vi "FP_Move Window to Control Location.vi"(8 "Error":errorcluster, 9 "Vi To Move Settings":T2={"Menu Bar"=FALSE, "Position"=enum."MID-CTR", "Decoration index"=0, "border(px)"=-2, "Point"={"Left"=0, "Top"=0}}, 10 "Point":T1, 11 "VI To Move":refnum<vi>) -> (0 "Error Out":errorcluster)   [LabVIEW 2020]
uses:
  TypeDefs_Utility/Cluster_FP on Point Set.ctl
  TypeDefs_Utility/ENUM RB_Pos_Quadrant Position.ctl
  TypeDefs_Utility/Cluster_Top Left position.ctl
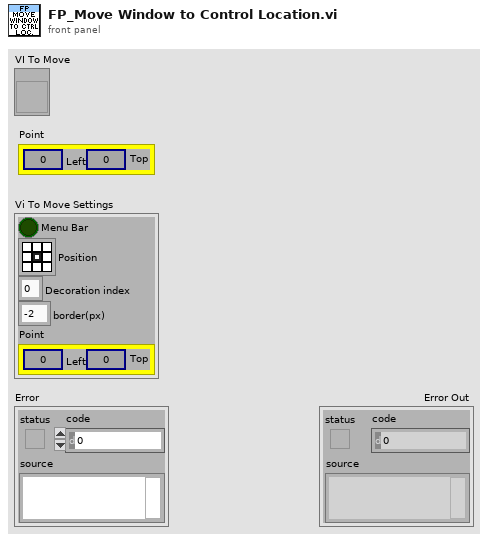
[diagram p1: front panel]
types:
  T1 = typedef "Cluster_Top Left position.ctl" = cluster{"Left":i32, "Top":i32}
  T2 = typedef "Cluster_FP on Point Set.ctl" = cluster{"Menu Bar":bool, "Position":T3, "Decoration index":i32, "border(px)":i32, "Point":T1}
  T3 = typedef "ENUM RB_Pos_Quadrant Position.ctl" = enum32{"LFT-TOP", "MID-TOP", "RGT-TOP", "LFT-CTR", "MID-CTR", "RGT-CTR", "LFT-BOT", "MID-BOT", "RGT-BOT"}
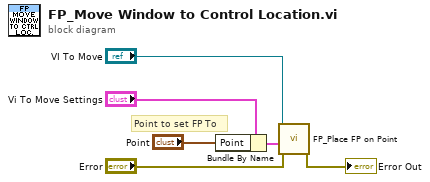
[diagram p0: block diagram]
diagram:
  # "Point to set FP To"
  n1 = Bundle By Name(cluster="Vi To Move Settings", "Point"="Point") -> (w4:T2)
  n2 = call "FP_Place FP on Point.vi"("Error"="Error", "FPSet"=w4, "VI Ref"="VI To Move") -> ("Error Out"=→"Error Out":errorcluster)  [unwired: 7 in, 1 out]
